vi "IVIS FRET_Analyze Data.vi"(6 "g":dbl=1.0 min=0.0, 8 "error in (no error)":errorcluster, 9 "Ordered ROI Type List":string[](array[string]), 10 "Ordered ROI Type Images":T5[](array[typedef]), 11 "[Frame Image Data]":T6[](array[typedef])) -> (0 "error out":errorcluster, 1 "Intensities":T1[](array[typedef]), 2 "Series Parameters & Coordinates":T2, 3 "[Coeffs & f_D E with SDVs]":T4[](array[typedef]))   [LabVIEW 2021]
uses:
  IVIS FRET_Frame Image Components.ctl
  <vilib>/vision/Image Controls.llb/IMAQ Image.ctl
  IVIS FRET_Frame Image Outputs.ctl
  IVIS FRET_Series Image Parameter & Coordinates.ctl
  Image/Image Point.ctl
  IVIS FRET_Frame Image Intensities.ctl
  IVIS FRET_Frame Image Components Data.ctl
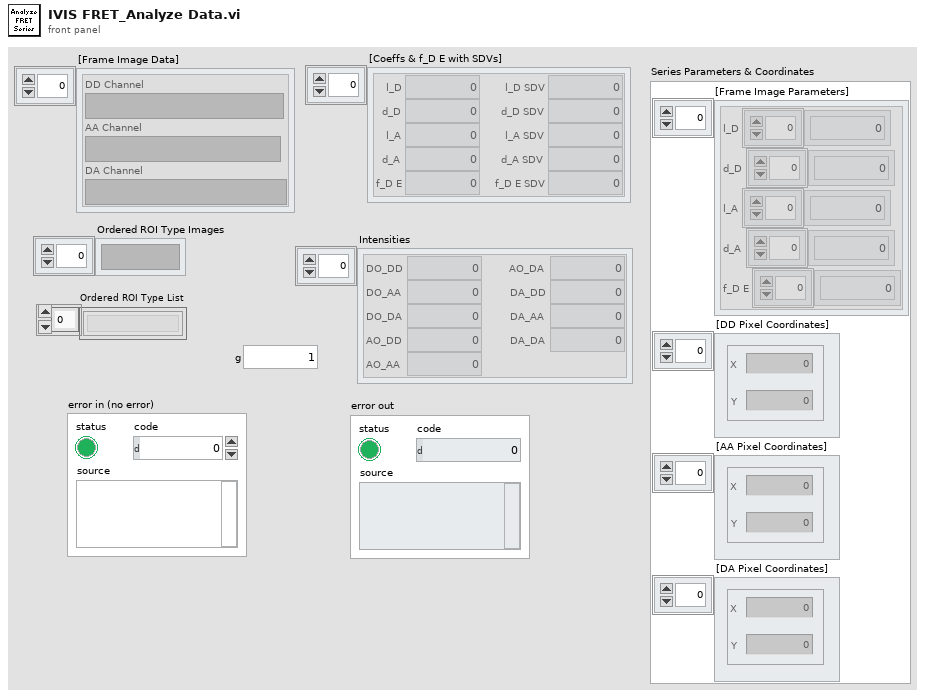
[diagram p1: front panel]
types:
  T1 = typedef "IVIS FRET_Frame Image Intensities.ctl" = cluster{"DO_DD":dbl, "DO_AA":dbl, "DO_DA":dbl, "AO_DD":dbl, "AO_AA":dbl, "AO_DA":dbl, "DA_DD":dbl, "DA_AA":dbl, "DA_DA":dbl}
  T2 = typedef "IVIS FRET_Series Image Parameter & Coordinates.ctl" = cluster{"[Frame Image Parameters]":cluster{"l_D":dbl[], "d_D":dbl[], "l_A":dbl[], "d_A":dbl[], "f_D E":dbl[]}[], "[DD Pixel Coordinates]":T3[], "[AA Pixel Coordinates]":T3[], "[DA Pixel Coordinates]":T3[]}
  T3 = typedef "Image Point.ctl" = cluster{"X":i32, "Y":i32}
  T4 = typedef "IVIS FRET_Frame Image Outputs.ctl" = cluster{"l_D":dbl, "l_D SDV":dbl, "d_D":dbl, "d_D SDV":dbl, "l_A":dbl, "l_A SDV":dbl, "d_A":dbl, "d_A SDV":dbl, "f_D E":dbl, "f_D E SDV":dbl}
  T5 = typedef "IMAQ Image.ctl" = refnum<image>
  T6 = typedef "IVIS FRET_Frame Image Components.ctl" = cluster{"DD Channel":T5, "AA Channel":T5, "DA Channel":T5}
  T7 = typedef "IVIS FRET_Frame Image Components Data.ctl" = cluster{"AO_DD":sgl[], "AO_AA":sgl[], "AO_DA":sgl[], "DO_DA":sgl[], "DO_AA":sgl[], "DO_DD":sgl[], "FRET_DA":sgl[], "FRET_AA":sgl[], "FRET_DD":sgl[], "[DD Pixel Coordinates]":T3[], "[AA Pixel Coordinates]":T3[], "[DA Pixel Coordinates]":T3[]}
  T8 = typedef "IVIS FRET_Frame Image Parameters.ctl" = cluster{"l_D":dbl[], "d_D":dbl[], "l_A":dbl[], "d_A":dbl[], "f_D E":dbl[]}
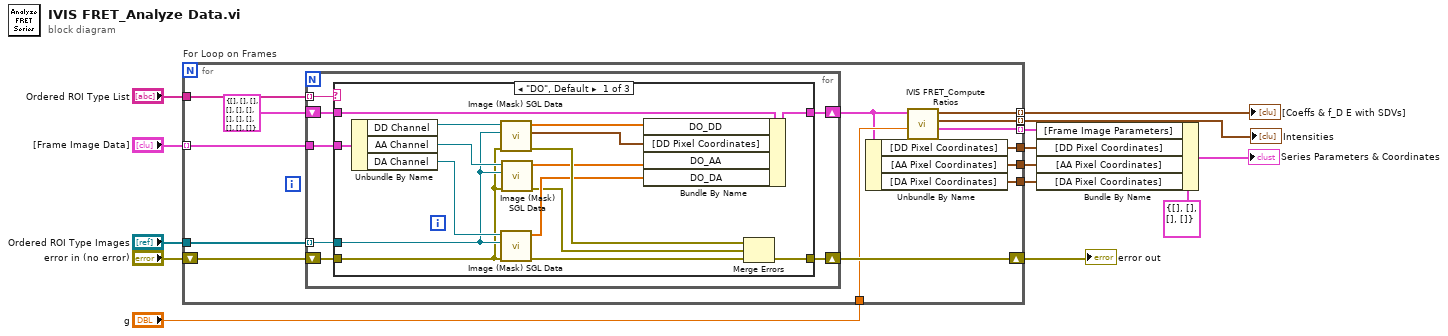
[diagram p0: block diagram]
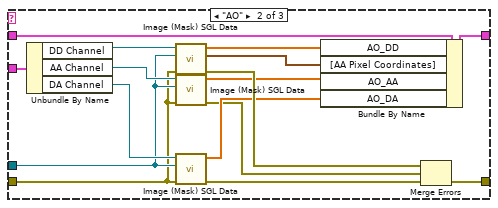
[diagram p2: hidden frame]
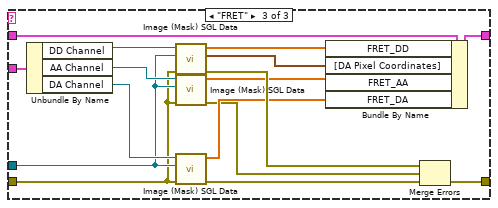
[diagram p3: hidden frame]
diagram:
  n1 = for "For Loop on Frames" {
    tunnel: "[Frame Image Data]" -> [w26] mode=indexing
    tunnel: "Ordered ROI Type Images" -> [w28]
    tunnel: "Ordered ROI Type List" -> [w27]
    shift-right: [w24] -> w10
    shift-left: "error in (no error)" -> [w25]
    tunnel: [w23] -> w8 mode=indexing
    tunnel: "g" -> [w22]
    tunnel: [w19] -> w4
    tunnel: [w18] -> w3
    tunnel: [w17] -> w2
    tunnel: [w16] -> w5 mode=indexing
    tunnel: [w15] -> w1 mode=indexing
    n2 = for {
      tunnel: w28 -> [w34] mode=indexing
      tunnel: w27 -> [w35] mode=indexing
      tunnel: w26 -> [w33]
      shift-right: [w31] -> w24
      shift-left: w25 -> [w32]
      shift-right: [w30] -> w20
      shift-left: T7 {"AO_DD"=[], "AO_AA"=[], "AO_DA"=[], "DO_DA"=[], "DO_AA"=[], "DO_DD"=[], "FRET_DA"=[], "FRET_AA"=[], "FRET_DD"=[], "[DD Pixel Coordinates]"=[], "[AA Pixel Coordinates]"=[], "[DA Pixel Coordinates]"=[]} ("Frame Image Components") -> [w29]
      n3 = case shown="\"DO\", Default" w35 {
        tunnel: w34 -> [w43 w59 w75]
        tunnel: w33 -> [w51 w67 w83]
        tunnel: w32 -> [w42 w58 w74]
        tunnel: [w40 w56 w72] -> w31
        tunnel: [w47 w63 w79] -> w30
        tunnel: w29 -> [w37 w53 w69]
        frame "DO", Default {
          n4 = Unbundle By Name(w51) -> ("DD Channel"=w50:T5, "AA Channel"=w46:T5, "DA Channel"=w44:T5)
          n5 = call "Image (Mask) SGL Data.vi"("error in (no error)"=w42, "Image Mask Refnum"=w43, "Src Image Refnum"=w50) -> ("error out"=w49:errorcluster, "[Pixel Coordinates]"=w36:T3[], "Pixel Values(Float)"=w48:sgl[])  [unwired: 3 in, 3 out]
          n6 = call "Image (Mask) SGL Data.vi"("error in (no error)"=w42, "Image Mask Refnum"=w43, "Src Image Refnum"=w44) -> ("error out"=w38:errorcluster, "Pixel Values(Float)"=w41:sgl[])  [unwired: 3 in, 4 out]
          n7 = call "Image (Mask) SGL Data.vi"("error in (no error)"=w42, "Image Mask Refnum"=w43, "Src Image Refnum"=w46) -> ("error out"=w39:errorcluster, "Pixel Values(Float)"=w45:sgl[])  [unwired: 3 in, 4 out]
          n8 = Bundle By Name(cluster=w37, "DO_DD"=w48, "[DD Pixel Coordinates]"=w36, "DO_AA"=w45, "DO_DA"=w41) -> (w47:T7)
          n9 = Merge Errors(w49, w39, w38) -> (w40:errorcluster)
        }
        frame "AO" {
          n10 = Unbundle By Name(w67) -> ("DD Channel"=w66:T5, "AA Channel"=w62:T5, "DA Channel"=w60:T5)
          n11 = call "Image (Mask) SGL Data.vi"("error in (no error)"=w58, "Image Mask Refnum"=w59, "Src Image Refnum"=w66) -> ("error out"=w65:errorcluster, "[Pixel Coordinates]"=w52:T3[], "Pixel Values(Float)"=w64:sgl[])  [unwired: 3 in, 3 out]
          n12 = call "Image (Mask) SGL Data.vi"("error in (no error)"=w58, "Image Mask Refnum"=w59, "Src Image Refnum"=w62) -> ("error out"=w55:errorcluster, "Pixel Values(Float)"=w61:sgl[])  [unwired: 3 in, 4 out]
          n13 = call "Image (Mask) SGL Data.vi"("error in (no error)"=w58, "Image Mask Refnum"=w59, "Src Image Refnum"=w60) -> ("error out"=w54:errorcluster, "Pixel Values(Float)"=w57:sgl[])  [unwired: 3 in, 4 out]
          n14 = Bundle By Name(cluster=w53, "AO_DD"=w64, "[AA Pixel Coordinates]"=w52, "AO_AA"=w61, "AO_DA"=w57) -> (w63:T7)
          n15 = Merge Errors(w65, w55, w54) -> (w56:errorcluster)
        }
        frame "FRET" {
          n16 = Unbundle By Name(w83) -> ("DD Channel"=w82:T5, "AA Channel"=w78:T5, "DA Channel"=w76:T5)
          n17 = call "Image (Mask) SGL Data.vi"("error in (no error)"=w74, "Image Mask Refnum"=w75, "Src Image Refnum"=w82) -> ("error out"=w81:errorcluster, "[Pixel Coordinates]"=w68:T3[], "Pixel Values(Float)"=w80:sgl[])  [unwired: 3 in, 3 out]
          n18 = call "Image (Mask) SGL Data.vi"("error in (no error)"=w74, "Image Mask Refnum"=w75, "Src Image Refnum"=w78) -> ("error out"=w71:errorcluster, "Pixel Values(Float)"=w77:sgl[])  [unwired: 3 in, 4 out]
          n19 = call "Image (Mask) SGL Data.vi"("error in (no error)"=w74, "Image Mask Refnum"=w75, "Src Image Refnum"=w76) -> ("error out"=w70:errorcluster, "Pixel Values(Float)"=w73:sgl[])  [unwired: 3 in, 4 out]
          n20 = Bundle By Name(cluster=w69, "FRET_DD"=w80, "[DA Pixel Coordinates]"=w68, "FRET_AA"=w77, "FRET_DA"=w73) -> (w79:T7)
          n21 = Merge Errors(w81, w71, w70) -> (w72:errorcluster)
        }
      }
    }
    n22 = Unbundle By Name(w20) -> ("[DD Pixel Coordinates]"=w19:T3[], "[AA Pixel Coordinates]"=w18:T3[], "[DA Pixel Coordinates]"=w17:T3[])
    n23 = call "IVIS FRET_Compute Ratios.vi"("g"=w22, "Frame Image Components"=w20) -> ("Frame Image Parameters"=w16:T8, "Frame Image Intensities"=w15:T1, "Frame Image Outputs"=w23:T4)  [unwired: 7 in]
  }
  "error out" <- w10
  "[Coeffs & f_D E with SDVs]" <- w8
  "Intensities" <- w1
  n24 = Bundle By Name(cluster=T2 {"[Frame Image Parameters]"=[], "[DD Pixel Coordinates]"=[], "[AA Pixel Coordinates]"=[], "[DA Pixel Coordinates]"=[]} ("Series Parameters & Coordinates"), "[Frame Image Parameters]"=w5, "[DD Pixel Coordinates]"=w4, "[AA Pixel Coordinates]"=w3, "[DA Pixel Coordinates]"=w2) -> (→"Series Parameters & Coordinates":T2)
